vi "SVI_PrettifyJSON_Caller.vi"(0 "File Path Control":path, 1 "Settings":T1={"Decimal Places"=3, "Array elements per line"=20}) -> (2 "standard output":string, 3 "return code":i32, 4 "standard error":string)   [LabVIEW 2014]
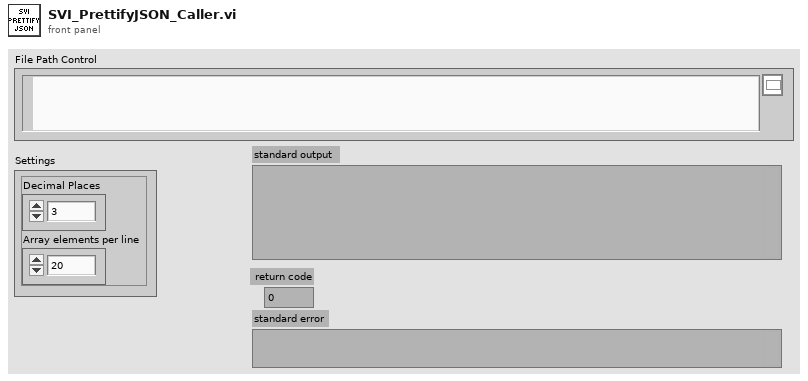
[diagram p1: front panel]
types:
  T1 = cluster{"Decimal Places":i32, "Array elements per line":i32}
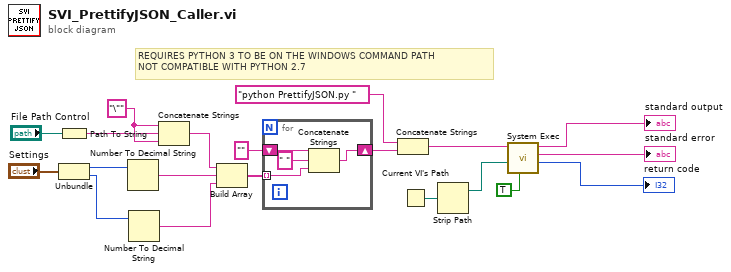
[diagram p0: block diagram]
diagram:
  w3 = "\"" ("string")
  # "REQUIRES PYTHON 3 TO BE ON THE WINDOWS COMMAND PATH\nNOT COMPATIBLE WITH PYTHON 2.7"
  n1 = Path To String(path="File Path Control") -> (string=w2:string)
  n2 = Unbundle("Settings") -> ("Decimal Places"=w5:i32, "Array elements per line"=w6:i32)
  n3 = Number To Decimal String(number=w5) -> (decimal integer string=w9:string)  [unwired: 1 in]
  n4 = Number To Decimal String(number=w6) -> (decimal integer string=w8:string)  [unwired: 1 in]
  n5 = Concatenate Strings(w3, w2, w3) -> (w1:string)
  n6 = Build Array(w1, w9, w8) -> (w14:string[])
  n7 = for {
    tunnel: w14 -> [w23] mode=indexing
    shift-right: [w21] -> w12
    shift-left: "" -> [w24]
    n8 = Concatenate Strings(w24, " " ("string"), w23) -> (w21:string)
  }
  n9 = Concatenate Strings("python PrettifyJSON.py " ("command line"), w12) -> (w13:string)
  n10 = Current VI's Path() -> (path=w17:path)
  n11 = Strip Path(path=w17) -> (stripped path=w16:path)  [unwired: 1 out]
  n12 = call <vilib>:"System Exec.vi"("run minimized? (F)"=TRUE, "working directory"=w16, "command line"=w13) -> ("return code"=→"return code":i32, "standard error"=→"standard error":string, "standard output"=→"standard output":string)  [unwired: 3 in, 3 out]
